vi "Add Album.vi"(8 "error in (no error)":errorcluster, 9 "Artist ID":i64, 10 "Name":string, 11 "SQLite Connection in":refnum<class "Connection.lvclass">) -> (0 "error out":errorcluster, 3 "SQLite Connection out":refnum<class "Connection.lvclass">)   [LabVIEW 2015]
doc: "Adds a new album to the database."
uses:
  <vilib>/drjdpowell/SQLite Library/SQL Connection/Connection.lvclass
  <vilib>/drjdpowell/SQLite Library/SQL Statement/SQL Statement.lvclass/SQL Statement.ctl
  <vilib>/drjdpowell/SQLite Library/SQL Statement/Bind Text.vi
  <vilib>/drjdpowell/SQLite Library/SQL Statement/Bind Integer.vi
  <vilib>/drjdpowell/SQLite Library/SQL Statement/Step.vi
  <vilib>/drjdpowell/SQLite Library/SQL Statement/Error Message.vi
  <vilib>/drjdpowell/SQLite Library/SQL Statement/SQL Statement.lvclass
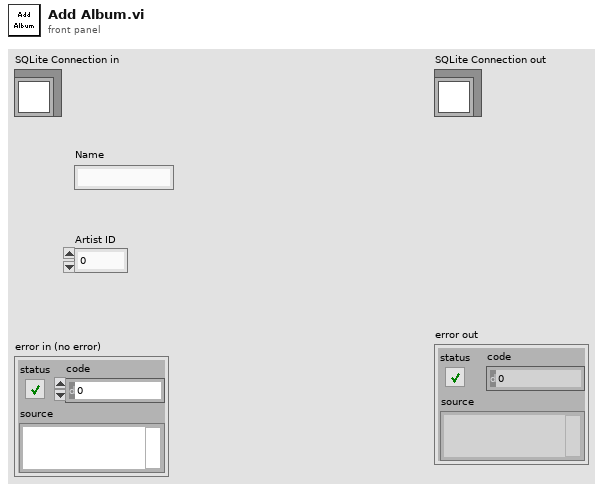
[diagram p1: front panel]
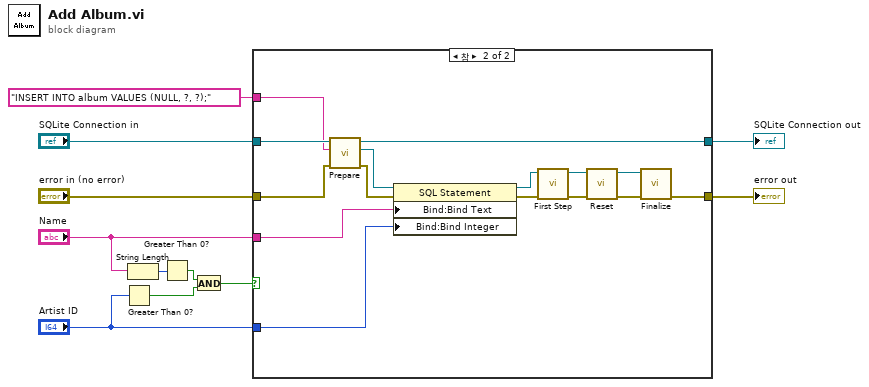
[diagram p0: block diagram]
diagram:
  n1 = Greater Than 0?(x="Artist ID") -> (x > 0?=w1:bool)
  n2 = String Length(string="Name") -> (length=w6:i32)
  n3 = Greater Than 0?(x=w6) -> (x > 0?=w3:bool)
  n4 = And(x=w3, y=w1) -> (x .and. y?=w2:bool)
  n5 = case shown="참" w2 {
    tunnel: "SQLite Connection in" -> [w13 w28]
    tunnel: "error in (no error)" -> [w12 w27]
    tunnel: "INSERT INTO album VALUES (NULL, ?, ?);" -> [_ w26]
    tunnel: [w13 w25] -> w8
    tunnel: [w12 w24] -> w7
    tunnel: "Name" -> [_ w15]
    tunnel: "Artist ID" -> [_ w14]
    frame False {
    }
    frame True {
      n6 = call <vilib>:"Prepare.vi"("error in (no error)"=w27, "SQL"=w26, "SQLite Connection in"=w28) -> ("error out"=w23:errorcluster, "SQL Statement"=w22:refnum<class "SQL Statement.lvclass">, "SQLite Connection"=w25:refnum<class "Connection.lvclass">)  [unwired: 4 in, 2 out]
      n7 = property class="SQL Statement"(reference=w22, error in=w23, "Bind:Bind Text"=w15, "Bind:Bind Integer"=w14) -> (reference out=w20:refnum<class "SQL Statement.lvclass">, error out=w21:errorcluster)
      n8 = call <vilib>:"First Step.vi"("error in (no error)"=w21, "SQL Statement in"=w20) -> ("error out"=w18:errorcluster, "SQL Statement"=w19:refnum<class "SQL Statement.lvclass">)  [unwired: 7 in, 1 out]
      n9 = call <vilib>:"Reset.vi"("error in (no error)"=w18, "SQL Statement in"=w19) -> ("error out"=w17:errorcluster, "SQL Statement"=w16:refnum<class "SQL Statement.lvclass">)  [unwired: 8 in]
      n10 = call <vilib>:"Finalize.vi"("error in (no error)"=w17, "SQL Statement in"=w16) -> ("error out"=w24:errorcluster)  [unwired: 9 in]
    }
  }
  "SQLite Connection out" <- w8
  "error out" <- w7
